vi "Pcre2PatternInfoSize8.vi"(8 "error in":errorcluster, 10 "What":u32 format="%.0x", 11 "pCode":u64 format="%.0x") -> (0 "error out":errorcluster, 1 "size":i32, 3 "pCode":u64 format="%.0x")   [LabVIEW 2021, in "libpcre2-8.lvlib"]
uses:
  libpcre2-8.lvlib
  libpcre2-8-x32.dll
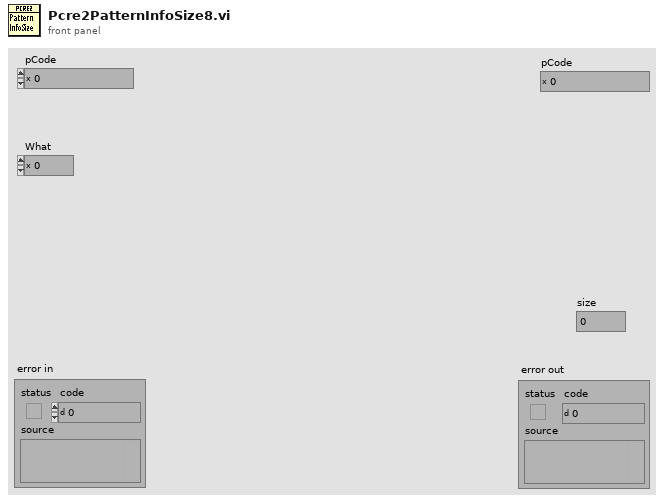
[diagram p1: front panel]
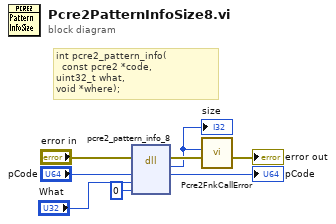
[diagram p0: block diagram]
diagram:
  # "int pcre2_pattern_info(\n  const pcre2 *code,\nuint32_t what,\nvoid *where);"
  n1 = dll-call lib="libpcre2-8-x*.dll" fn="pcre2_pattern_info_8"(error in="error in", "code"="pCode", "what"="What", "where"=u64 0) -> (error out=w3:errorcluster, "return type"=w1:i32, "code"=→"pCode":u64)  [unwired: 4 in, 1 out]
  "size" <- w1
  n2 = call "Pcre2FnkCallError.vi"("error in"=w3, "ErrorCode"=w1) -> ("error out"=→"error out":errorcluster)  [unwired: 9 in]
